vi "EXE Test.vi"() -> ()   [LabVIEW 2009]
uses:
  Tests/MyFirstTest/MyFirstTest.lvclass
  Programmatic API/Run Tests (Test Object).vi
  Programmatic API/VI Tester API.lvlib
panel:
  out "error out":errorcluster
  out "successful?":bool
  out "test details":string
  # "API Test"
  # "GUI Test"
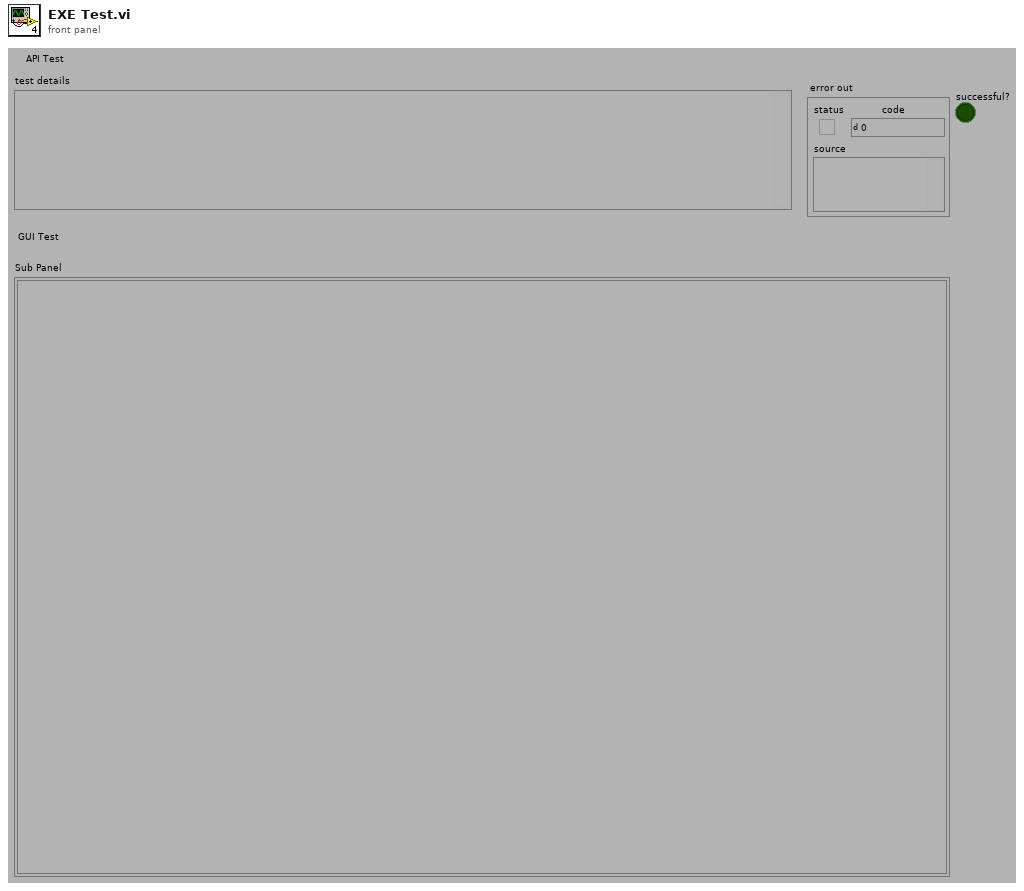
[diagram p1: front panel]
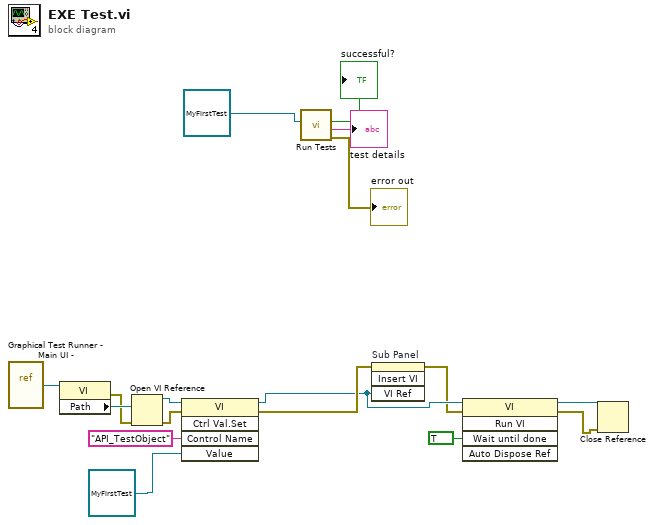
[diagram p0: block diagram]
diagram:
  n1 = vi-ref "Graphical Test Runner - Main UI - .vi"() -> (w13:refnum<vi>)
  n2 = property class="VI"(reference=w13) -> (error out=w1:errorcluster, "Path"=w12:path)  [unwired: 1 in, 1 out]
  n3 = Open VI Reference(vi path=w12, error in (no error)=w1) -> (vi reference=w11:refnum<vi>, error out=w2:errorcluster)  [unwired: 4 in]
  n4 = invoke class="VI" method="Ctrl Val.Set"(reference=w11, error in=w2, "Control Name"="API_TestObject", "Value"=refnum<class "MyFirstTest.lvclass"> refnum ("MyFirstTest.lvclass")) -> (reference out=w7:refnum<vi>, error out=w8:errorcluster)  [unwired: 1 in, 3 out]
  n5 = call-poly "Run Tests.vi"("Test"=refnum<class "MyFirstTest.lvclass"> refnum ("MyFirstTest.lvclass")) -> ("error out"=→"error out":errorcluster, "test details"=→"test details":string, "successful?"=→"successful?":bool)  [unwired: 8 in]
  n6 = invoke on="Sub Panel" class="SubPanel" method="Insert VI"(error in=w8, "VI Ref"=w7) -> (error out=w3:errorcluster)  [unwired: 2 in, 3 out]
  n7 = invoke class="VI" method="Run VI"(reference=w7, error in=w3, "Wait until done"=TRUE ("Wait Until Done")) -> (reference out=w5:refnum<vi>, error out=w4:errorcluster)  [unwired: 2 in, 3 out]
  n8 = Close Reference(reference=w5, error in (no error)=w4) -> ()  [unwired: 1 out]
